vi "Check Internet Access Status.vi"(8 "Error In":errorcluster, 10 "Warnings in":T5[](array[typedef]), 11 "Install LV Data":T1={"SSH Session"=refnum, "Status Log"="", "Detailed Log"="", "Credentials"={"Hostname or IP"="192.168.7.2", "Username"="root", "Password"=""}, "Target Info"={"OS Version"="", "CPU"="", "Systemd Version"="", "Internet Access"=FALSE, "Device Type"="", "LV Installed Ver"="", "LV Available Ver"="", "LV Upgrade Available"=FALSE, "Hostname"="", "NIC Info"=[]}, "Reboot Required?"=FALSE}) -> (0 "Error Out":errorcluster, 2 "Warnings out":T5[](array[typedef]), 3 "Install LV Data":T1={"SSH Session"=refnum, "Status Log"="", "Detailed Log"="", "Credentials"={"Hostname or IP"="192.168.7.2", "Username"="root", "Password"=""}, "Target Info"={"OS Version"="", "CPU"="", "Systemd Version"="", "Internet Access"=FALSE, "Device Type"="", "LV Installed Ver"="", "LV Available Ver"="", "LV Upgrade Available"=FALSE, "Hostname"="", "NIC Info"=[]}, "Reboot Required?"=FALSE})   [LabVIEW 2020, in "LMH-LINX.lvlib"]
uses:
  LMH-LINX.lvlib
  Install LV Data.ctl
  Target Info.ctl
  NIC Info.ctl
  NIC Mode.ctl
  Target Compatibility Warnings.ctl
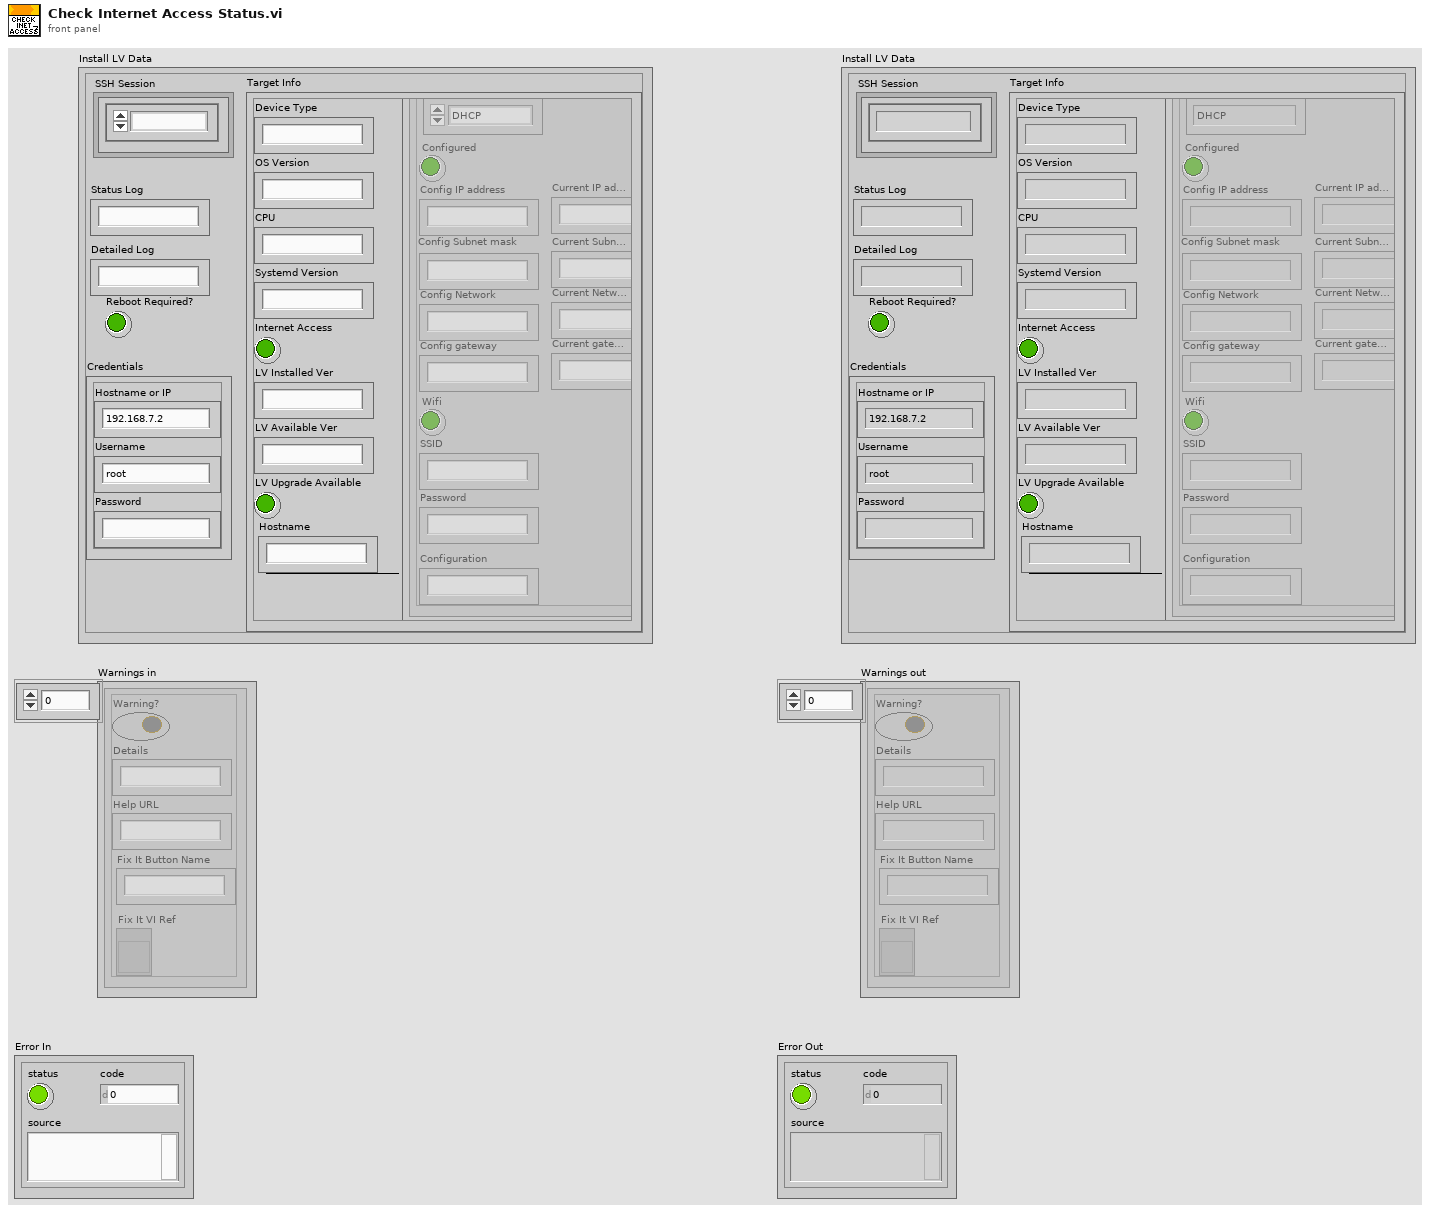
[diagram p1: front panel]
types:
  T1 = typedef "LMH-LINX.lvlib/Install LV Data.ctl" = cluster{"SSH Session":refnum<k1>, "Status Log":string, "Detailed Log":string, "Credentials":cluster{"Hostname or IP":string, "Username":string, "Password":string}, "Target Info":T2, "Reboot Required?":bool}
  T2 = typedef "LMH-LINX.lvlib/Target Info.ctl" = cluster{"OS Version":string, "CPU":string, "Systemd Version":string, "Internet Access":bool, "Device Type":string, "LV Installed Ver":string, "LV Available Ver":string, "LV Upgrade Available":bool, "Hostname":string, "NIC Info":T3[]}
  T3 = typedef "LMH-LINX.lvlib/NIC Info.ctl" = cluster{"Name":string, "NIC Mode":T4, "Configured":bool, "Config IP address":string, "Config Subnet mask":string, "Config Network":string, "Config gateway":string, "Wifi":bool, "SSID":string, "Password":string, "Configuration":string, "Current IP address":string, "Current Subnet mask":string, "Current gateway":string, "Current Network":string}
  T4 = typedef "LMH-LINX.lvlib/NIC Mode.ctl" = enum16{"DHCP", "Static", "Loopback"}
  T5 = typedef "LMH-LINX.lvlib/Target Compatibility Warnings.ctl" = cluster{"Warning?":bool, "Details":string, "Help URL":string, "Fix It Button Name":string, "Fix It VI Ref":refnum<vi>}
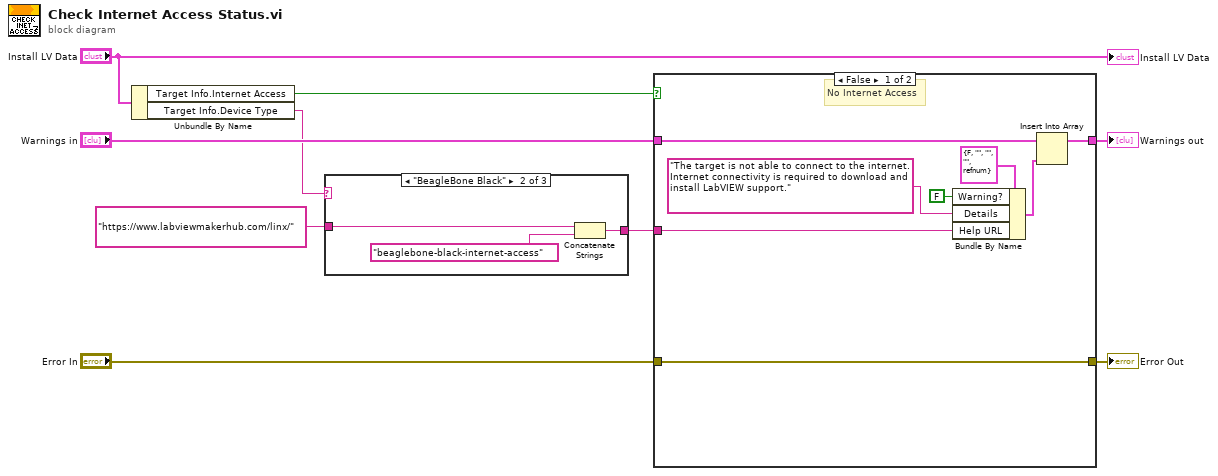
[diagram p0: block diagram]
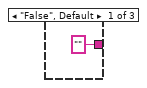
[diagram p2: hidden frame]
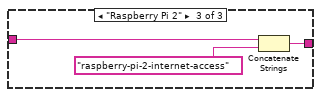
[diagram p3: hidden frame]
diagram:
  n1 = Unbundle By Name("Install LV Data") -> ("Target Info.Internet Access"=w1:bool, "Target Info.Device Type"=w6:string)
  n2 = case shown="\"BeagleBone Black\"" w6 {
    tunnel: ["" w12 w15] -> w2
    tunnel: "https://www.labviewmakerhub.com/linx/" -> [_ w11 w14]
    frame "False", Default {
    }
    frame "BeagleBone Black" {
      n3 = Concatenate Strings(w11, "beaglebone-black-internet-access" ("string")) -> (w12:string)
    }
    frame "Raspberry Pi 2" {
      n4 = Concatenate Strings(w14, "raspberry-pi-2-internet-access" ("string")) -> (w15:string)
    }
  }
  n5 = case shown="False" w1 {
    tunnel: "Warnings in" -> [w21 w26]
    tunnel: [w19 w26] -> w7
    tunnel: w2 -> [w18 _]
    tunnel: "Error In" -> [w17 w25]
    tunnel: [w17 w25] -> w4
    frame False {
      # "No Internet Access"
      n6 = Bundle By Name(cluster=T5 {"Warning?"=FALSE, "Details"="", "Help URL"="", "Fix It Button Name"="", "Fix It VI Ref"=refnum} ("Target Compatibility Warnings"), "Warning?"=FALSE ("Can Continue?"), "Details"="The target is not able to connect to the internet.  Internet connectivity is required to download and install LabVIEW support.", "Help URL"=w18) -> (w22:T5)
      n7 = Insert Into Array(array=w21, new element=w22) -> (w19:T5[])  [unwired: 1 in]
    }
    frame True {
      # "Internet Access"
    }
  }
  "Warnings out" <- w7
  "Error Out" <- w4
  "Install LV Data" <- "Install LV Data"
